vi "Acitvate Node.vi"(8 "error in (no error)":errorcluster, 10 "Active Node(\"\")":string, 11 "TREE in":refnum<class "MyTreeAPI.lvclass">) -> (0 "error out":errorcluster, 3 "TREE out":refnum<class "MyTreeAPI.lvclass">)   [LabVIEW 2015, in "MyTreeAPI.lvclass"]
uses:
  MyTreeAPI.lvclass
  MyTreeAPI.lvclass/MyTreeAPI.ctl
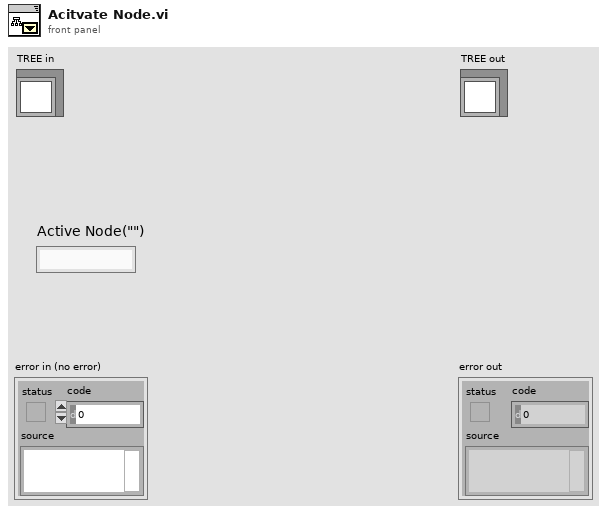
[diagram p1: front panel]
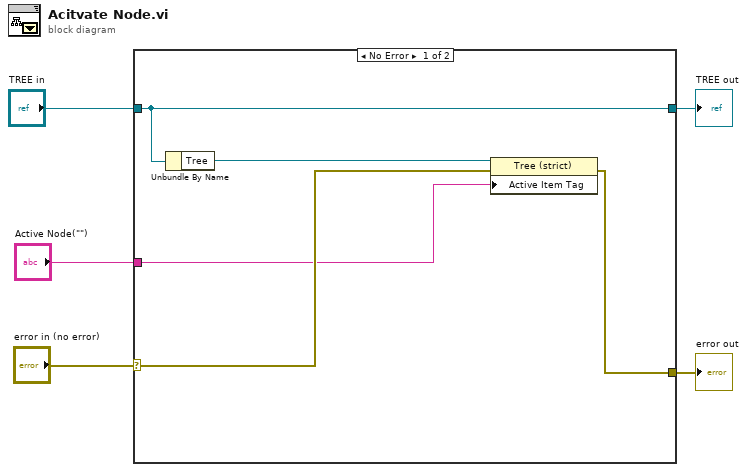
[diagram p0: block diagram]
diagram:
  n1 = case shown="No Error" "error in (no error)" {
    selector: "error in (no error)" -> [w7 w12]
    tunnel: [w9 w12] -> w4
    tunnel: [w10 w11] -> w2
    tunnel: "TREE in" -> [w10 w11]
    tunnel: "Active Node(\"\")" -> [w6 _]
    frame No Error {
      n2 = Unbundle By Name(w10) -> ("Tree"=w8:refnum<vi>)
      n3 = property class="Tree (strict)"(reference=w8, error in=w7, "Active Item Tag"=w6) -> (error out=w9:errorcluster)  [unwired: 1 out]
    }
    frame Error {
    }
  }
  "error out" <- w4
  "TREE out" <- w2
